vi "CTRE_Phoenix_CANCoder_GetFeedbackCoefficient.vi"(6 "timeoutMs":i32, 8 "error in":errorcluster, 11 "CTRE_CANcoder_DeviceRef":T1) -> (0 "error out":errorcluster, 2 "Feedback Coefficient":dbl format="%.2f", 3 "CTRE_CANcoder_DeviceRef":T1)   [LabVIEW 2020]
doc: "Returns the absolute position of the CANcoder."
uses:
  <vilib>/Rock Robotics/WPI/ThirdParty/Phoenix-LabVIEW/CANCoder/Controls/CTRE_Phoenix_CANcoder_DeviceRef.ctl
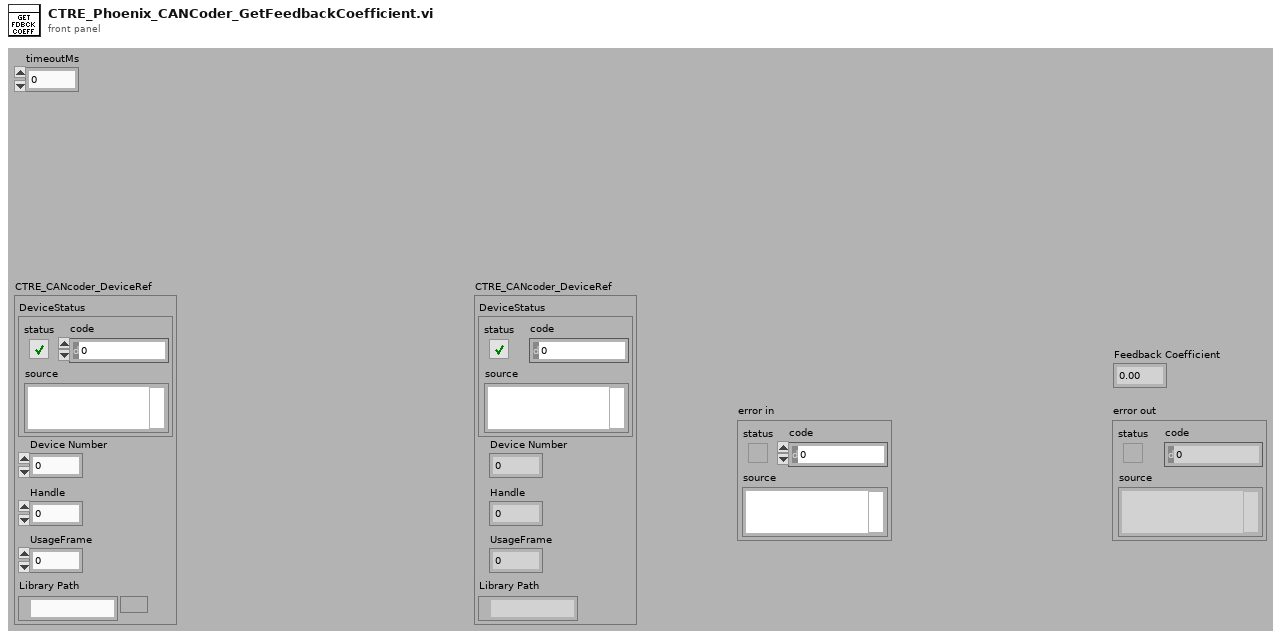
[diagram p1: front panel]
types:
  T1 = typedef "CTRE_Phoenix_CANcoder_DeviceRef.ctl" = cluster{"DeviceStatus":errorcluster, "Device Number":u8, "Handle":u64, "UsageFrame":u32, "Library Path":path}
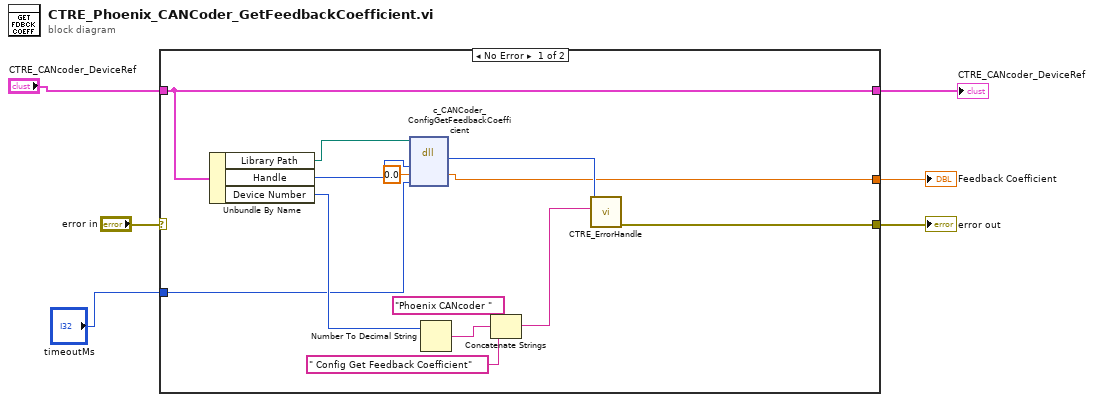
[diagram p0: block diagram]
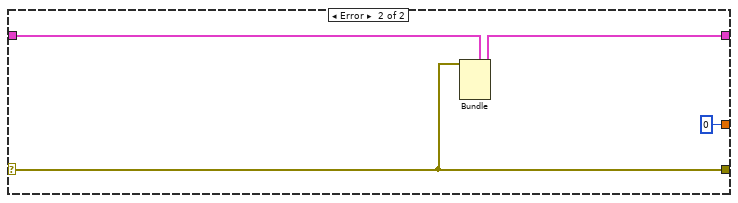
[diagram p2: hidden frame]
diagram:
  n1 = case shown="No Error" "error in" {
    selector: "error in" -> [_ w22]
    tunnel: "CTRE_CANcoder_DeviceRef" -> [w12 w23]
    tunnel: [w19 w22] -> w6
    tunnel: [w12 w21] -> w2
    tunnel: [w13 0 ("percentOutput")] -> w4
    tunnel: "timeoutMs" -> [w8 _]
    frame No Error {
      n2 = Unbundle By Name(w12) -> ("Library Path"=w10:path, "Handle"=w9:u64, "Device Number"=w11:u8)
      n3 = dll-call lib="?" fn="c_CANCoder_ConfigGetFeedbackCoefficient"(path in=w10, "handle"=w9, "feedbackCoefficient"=0.0 ("offsetDegrees"), "timeoutMs"=w8) -> ("return type"=w15:i32, "feedbackCoefficient"=w13:dbl)  [unwired: 4 in, 2 out]
      n4 = Number To Decimal String(number=w11) -> (decimal integer string=w17:string)  [unwired: 1 in]
      n5 = Concatenate Strings("Phoenix CANcoder " ("string"), w17, " Config Get Feedback Coefficient" ("string")) -> (w14:string)
      n6 = call <vilib>:"CTRE_ErrorHandle.vi"("origin"=w14, "code"=w15) -> ("error out"=w19:errorcluster)  [unwired: 9 in]
    }
    frame Error {
      n7 = Bundle(cluster=w23, "DeviceStatus"=w22) -> (w21:T1)  [unwired: 4 in]
    }
  }
  "Feedback Coefficient" <- w4
  "error out" <- w6
  "CTRE_CANcoder_DeviceRef" <- w2
